vi "Aotunomous constants.vi"() -> (4 "Throttle":dbl, 6 "Wanted Angle":dbl, 8 "Time Of Trigger (S)":dbl, 10 "Time Of Conveyer Belt (S)":dbl, 15 "Power Of Conveyer Belt":dbl)   [LabVIEW 2012]
panel:
  in  "Power Of Conveyer Belt":dbl
  in  "Time Of Conveyer Belt (S)":dbl
  in  "Time Of Trigger (S)":dbl
  in  "Wanted Angle":dbl
  in  "Throttle":dbl
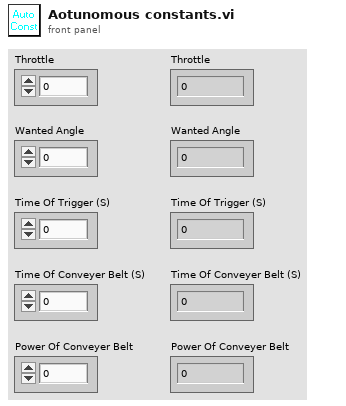
[diagram p1: front panel]
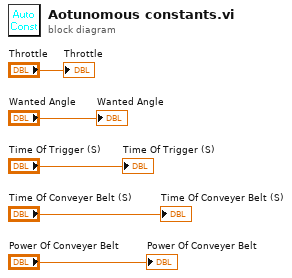
[diagram p0: block diagram]
diagram:
  "Throttle" <- "Throttle"
  "Wanted Angle" <- "Wanted Angle"
  "Time Of Trigger (S)" <- "Time Of Trigger (S)"
  "Time Of Conveyer Belt (S)" <- "Time Of Conveyer Belt (S)"
  "Power Of Conveyer Belt" <- "Power Of Conveyer Belt"
